vi "Calc overheat ratio.vi"(1 "Bridge ratio":dbl=1.0, 2 "Rset (ohm)":dbl=6.2, 3 "RL (ohm)":dbl=0.5, 4 "R0 (ohm)":dbl=3.5) -> (0 "Overheat ratio (Rw/R0)":dbl=1.6285714285714286)   [LabVIEW 2021]
doc: "Calculate the overheat ratio (Rw / R0) from the variable wire parameters and fixed bridge parameters.\nPN 06-NOV-23."
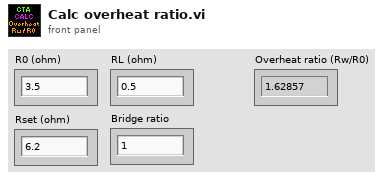
[diagram p1: front panel]
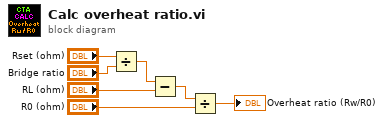
[diagram p0: block diagram]
diagram:
  n1 = Divide(x="Rset (ohm)", y="Bridge ratio") -> (x/y=w1:dbl)
  n2 = Subtract(x=w1, y="RL (ohm)") -> (x-y=w4:dbl)
  n3 = Divide(x=w4, y="R0 (ohm)") -> (x/y=→"Overheat ratio (Rw/R0)":dbl)
